vi "Dynamic Configure Distance Sensors.vi"(0 "Device ID":T1(ring), 1 "D1_Tolerance":u32=20, 2 "Distance Sensor Mode":enum32{"Voltage", "Distance"}(ring)=enum."Distance", 5 "D1_Level":u32=512, 7 "D1_Repetition_Value":u32=3, 9 "D2_Tolerance":u32=20, 11 "error in":errorcluster, 12 "D2_Level":u32=512, 13 "D2_Repetition_Value":u32=3) -> (4 "Device ID Out":T1(ring), 15 "error out":errorcluster)   [LabVIEW 2010]
doc: "You can only configure the digital distance sensors before the transfer area is started. This vi stops any existing transfer area for the specified Device ID, configures the digital distance sensors, and restarts the transfer area. Currently, the Robo Interface is the only Interface Type to support digital distance sensors.\n\nCaution: If any other VI trys to access the transfer area when this VI is running, you will most likely get an error. Program accordingly."
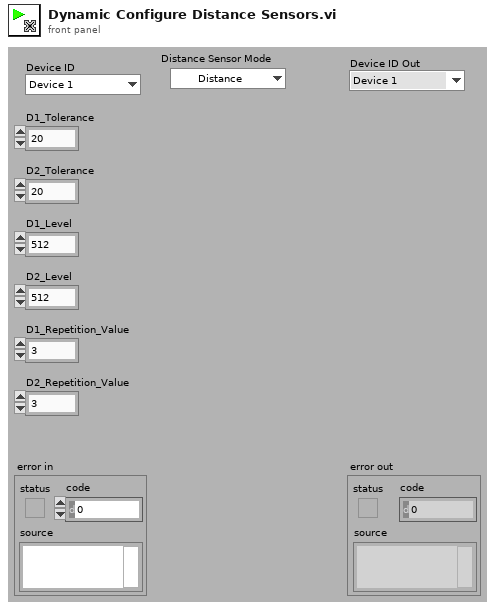
[diagram p1: front panel]
types:
  T1 = enum16{"Device 1", "Device 2", "Device 3", "Device 4", "Device 5", "Device 6", "Device 7", "Device 8"}
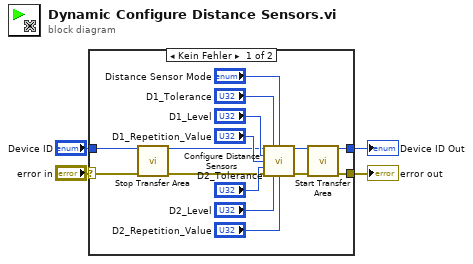
[diagram p0: block diagram]
diagram:
  n1 = case shown="Kein Fehler" "error in" {
    selector: "error in" -> [w12 w21]
    tunnel: [w5 w21] -> w3
    tunnel: "Device ID" -> [w10 w20]
    tunnel: [w7 w20] -> w1
    frame No Error {
      n2 = call "Stop Transfer Area.vi"("Device ID"=w10, "error in"=w12) -> ("Device ID Out"=w9:T1, "error out"=w11:errorcluster)  [unwired: 12 out]
      n3 = call "Configure Distance Sensors.vi"("Device ID"=w9, "D1_Tolerance"="D1_Tolerance", "Distance Sensor Mode"="Distance Sensor Mode", "D1_Level"="D1_Level", "D1_Repetition_Value"="D1_Repetition_Value", "D2_Tolerance"="D2_Tolerance", "error in"=w11, "D2_Level"="D2_Level", "D2_Repetition_Value"="D2_Repetition_Value") -> ("Device ID Out"=w8:T1, "error out"=w6:errorcluster)  [unwired: 5 out]
      n4 = call "Start Transfer Area.vi"("Device ID"=w8, "error in"=w6) -> ("Device ID Out"=w7:T1, "error out"=w5:errorcluster)  [unwired: 12 out]
    }
    frame Error {
    }
  }
  "error out" <- w3
  "Device ID Out" <- w1
